vi "nominal ingest mcap set ignore invalid topics.vi"(8 "error in (no error)":errorcluster, 10 "ignore":bool, 11 "staging":i32) -> (0 "error out":errorcluster, 3 "function return":i32)   [LabVIEW 2020, in "client.lvlib"]
doc: "int32_t nominal_ingest_mcap_set_ignore_invalid_topics(int32_t staging, bool ignore);"
uses:
  client.lvlib
  bin/nominalClient_64.dll
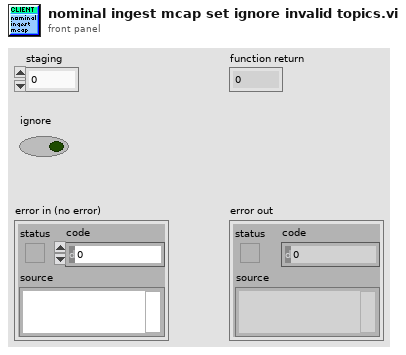
[diagram p1: front panel]
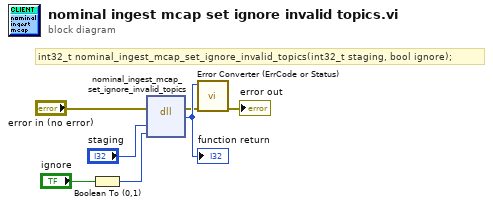
[diagram p0: block diagram]
diagram:
  # "int32_t nominal_ingest_mcap_set_ignore_invalid_topics(int32_t staging, bool ignore);"
  n1 = Boolean To (0,1)(Boolean="ignore") -> (0, 1=w4:i16)
  n2 = dll-call lib="C:/code/labview-client-rs/lv_src/bin/nominalClient_*.*" fn="nominal_ingest_mcap_set_ignore_invalid_topics"(error in="error in (no error)", "staging"="staging", "ignore"=w4) -> (error out=w2:errorcluster, w7:i32)  [unwired: 4 in, 1 out]
  "function return" <- w7
  n3 = call "Error Converter (ErrCode or Status).vi"("error in (no error)"=w2, "error code"=w7) -> ("error out"=→"error out":errorcluster)  [unwired: 9 in]
